vi "Hola Mundo Serial.vi"() -> ()   [LabVIEW 2020]
uses:
  <vilib>/Instr/_visa.llb/VISA Configure Serial Port (Instr).vi
panel:
  out "RX":string
  in  "tx send":string
  in  "Puerto COM":refnum<visa-resource-name>
  in  "Paridad":enum16{"None", "Odd", "Even", "Mark", "Space"}(ring)
  in  "Baudios":u32=9600
  in  "stop":bool
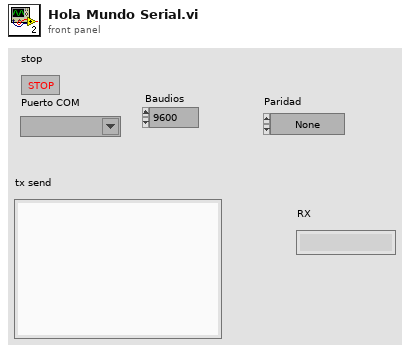
[diagram p1: front panel]
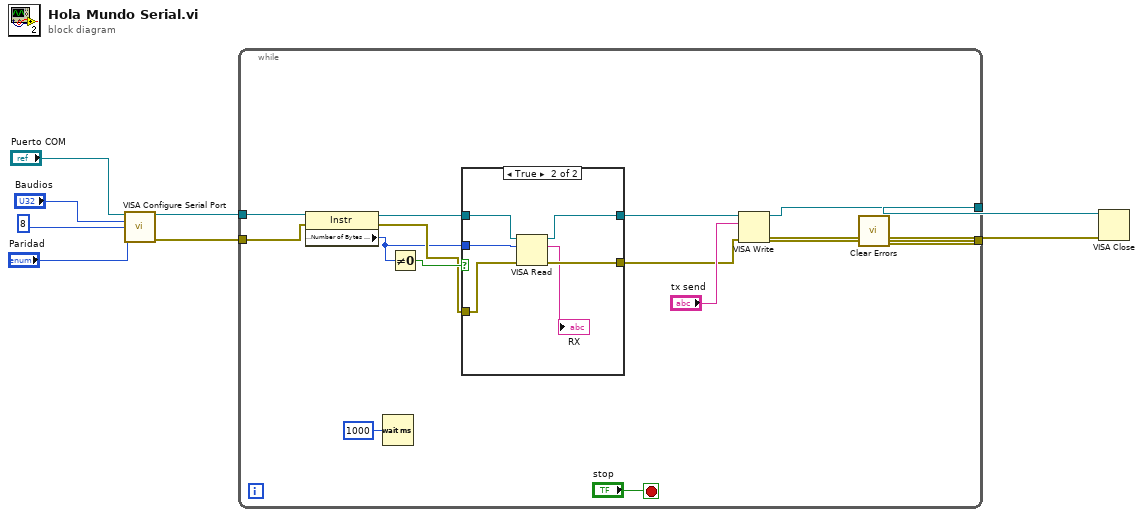
[diagram p0: block diagram]
diagram:
  n1 = call-poly "VISA Configure Serial Port"("VISA resource name"="Puerto COM", "baud rate (9600)"="Baudios", "data bits (8)"=u16 8, "parity (0:none)"="Paridad") -> ("VISA resource name out"=w4:refnum<visa-resource-name>, "error out"=w3:errorcluster)  [unwired: 10 in]
  n2 = while {
    tunnel: w4 -> [w16]
    tunnel: w3 -> [w15]
    tunnel: [w17] -> w2
    tunnel: [w18] -> w1
    stop <- "stop" stop-if-true
    n3 = property class="Instr"(reference=w16, error in=w15) -> (reference out=w13:refnum<visa-resource-name>, error out=w12:errorcluster, "Serial Settings:Number of Bytes at Serial Port"=w11:u32)
    n4 = Wait (ms)(milliseconds to wait=u32 1000) -> ()  [unwired: 1 out]
    n5 = Not Equal To 0?(x=w11) -> (x != 0?=w14:bool)
    n6 = case shown="True" w14 {
      tunnel: w13 -> [w24 w30]
      tunnel: w12 -> [w23 w29]
      tunnel: w11 -> [_ w28]
      tunnel: [w24 w27] -> w10
      tunnel: [w23 w26] -> w9
      frame False {
      }
      frame True {
        n7 = VISA Read(VISA resource name=w30, byte count=w28, error in (no error)=w29) -> (VISA resource name out=w27:refnum<visa-resource-name>, read buffer=→"RX":string, error out=w26:errorcluster)  [unwired: 1 out]
      }
    }
    n8 = VISA Write(VISA resource name=w10, write buffer="tx send", error in (no error)=w9) -> (VISA resource name out=w17:refnum<visa-resource-name>, error out=w19:errorcluster)  [unwired: 1 out]
    n9 = call <vilib>:"Clear Errors.vi"("error in (no error)"=w19) -> ("error out"=w18:errorcluster)  [unwired: 5 in, 1 out]
  }
  n10 = VISA Close(VISA resource name=w2, error in (no error)=w1) -> ()  [unwired: 1 out]
